vi "WGR.vi"(0 "System no.":i32=1 min=1 max=4 step=1, 5 "error in":errorcluster) -> (19 "error out":errorcluster)   [LabVIEW 2026]
doc: "Starts a new recording.\n\nC-413: Use DRC to configure data recording. Recording ends when the record table content has reached the maximum number of points (4096 in total).\n\nC-886: Recording ends when the record table content has reached the maximum number of points (8192 per table).\n\nC-887: Use DRC to configure data recording. Recording ends when the record table content has reached the maximum number of points (4 Million in total). \n\nC-891: Use DRC to configure data recording. Recording ends when the record table content has reached the maximum number of points (16384 in total).\n\nE-517, E-518: Use DRC to configure data recording. Recording ends when the record table content has reached the maximum number of points (8,192 in total). If more than one wave generator is running, recording starts at the waveform start point which occurs first.\n\nE-709: Use DRC to configure data recording. Recording ends when the record table content has reached the maximum number of points (4096 in total).\n\nE-712: Use DRC to configure data recording. Recording ends when the record table content has reached the maximum number of points (262,144 in total).\n\nE-725, E-727: Use DRC to configure data recording. Recording ends when the record table content has reached the maximum number of points (262,144 in total).\n\nE-753: Use DRC to configure data recording. Recording ends when the record table content has reached the maximum number of points (65,536 in total).\n\nE-754: Use DRC to configure data recording. Recording ends when the record table content has reached the maximum number of points (1,048,576 in total).\n\nE-761: Recording will be started for all recorder tables when the wave generator is running for an arbitraray axis. The assignment of axis and data sources to the recorder tables is as follows:\ntable 1: axis 1 actual position\ntable 2: axis 2 actual position\ntable 3: axis 3 actual position\ntable 4: analog input voltage (same value as read with TAV?.vi, i.e. contains gain and offset for the analog input, see E-761 user manual). Recording starts always with the next start point of the waveform, i.e. there might be a short delay between sending WGR and the start of the record. If more than one wave generator is running, recording starts at the waveform start point which occurs first. Recording ends when the record table content has reached the maximum number of points (8192 per table)."
panel:
  # "Starts a new recording."
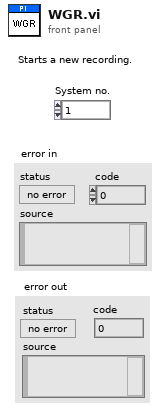
[diagram p1: front panel]
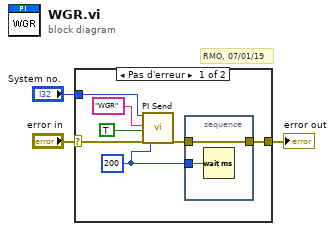
[diagram p0: block diagram]
diagram:
  # "RMO, 07/01/19"
  n1 = case shown="Pas d'erreur" "error in" {
    selector: "error in" -> [w4 w13]
    tunnel: [w6 w13] -> w3
    tunnel: "System no." -> [w7 _]
    frame No Error {
      w5 = u32 200 ("milliseconds to wait")
      n2 = call "PI Send.vi"("System no."=w7, "String to send"="WGR", "Attach termination char.?"=TRUE ("Attach Linefeed?"), "error in"=w4, "Delay before error check (ms)"=w5) -> ("error out"=w9:errorcluster)  [unwired: 1 in, 13 out]
      n3 = stacked-sequence {
        tunnel: w9 -> [w12]
        tunnel: [w12] -> w6
        tunnel: w5 -> [w11]
        frame #0 {
          n4 = Wait (ms)(milliseconds to wait=w11) -> ()  [unwired: 1 out]
        }
      }
    }
    frame Error {
    }
  }
  "error out" <- w3
